vi "信号处理素材.vi"() -> ()   [LabVIEW 2018]
uses:
  <vilib>/Analysis/2dsp.llb/Upsample (DBL).vi
  <vilib>/Analysis/3filter.llb/Equi-Ripple LowPass (DBL).vi
  <vilib>/Analysis/NI_AALBase.lvlib
  <vilib>/Analysis/NI_AALPro.lvlib
panel:
  out "波形图 7":T1(graph)
  out "波形图 6":dbl[](graph)
  in  "sampling freq: fs":dbl=1.0 caption="采样频率:fs" format="%0.2f"
  in  "stop freq":dbl=0.25 caption="阻带截止频率" format="%0.2f"
  in  "pass freq":dbl=0.2 caption="通带截止频率" format="%0.2f"
  out "波形图 5":T1(graph)
  out "波形图 4":dbl[](graph)
  in  "upsampling factor":i32=1 caption="升采样因子"
  out "波形图 3":T1(graph)
  out "波形图 2":dbl[](graph)
  out "phase out":dbl caption="相位输出" format="%0.2e"
  in  "phase in":dbl caption="相位输入" format="%0.2f"
  in  "duty cycle (%)":dbl=50.0 caption="占空比(%)" format="%0.2f"
  in  "frequency":dbl=0.0078125 caption="频率" format="%.4f"
  in  "amplitude 3":dbl=1.0 caption="幅值" format="%0.2f"
  in  "samples 3":i32=128 caption="采样"
  in  "samples 2":i32=128 caption="采样"
  in  "amplitude 2":dbl=1.0 caption="幅值" format="%0.2f"
  out "波形图":dbl[](graph)
  in  "samples":i32=128 caption="采样"
  in  "amplitude":dbl=1.0 caption="幅值" format="%0.2f"
  in  "phase(degrees)":dbl caption="相位（度）" format="%0.2f"
  in  "cycles":dbl=1.0 caption="周期" format="%0.2f"
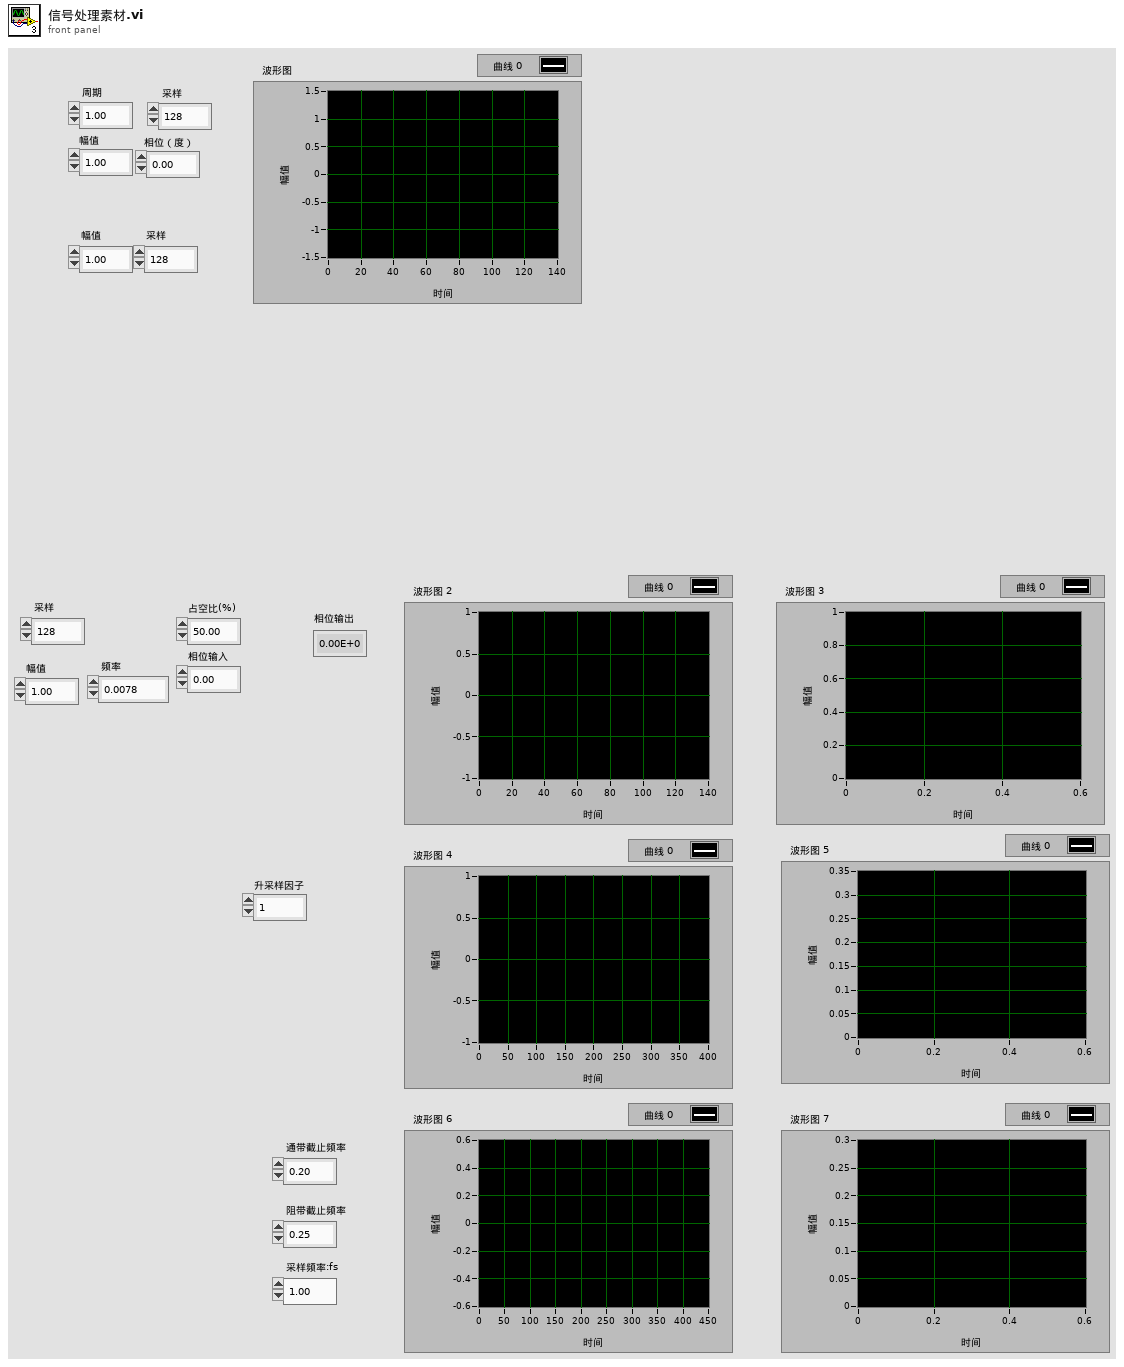
[diagram p1: front panel]
types:
  T1 = cluster{i32, "df":dbl, "Amp Spectrum Mag (Vrms)":dbl[]}
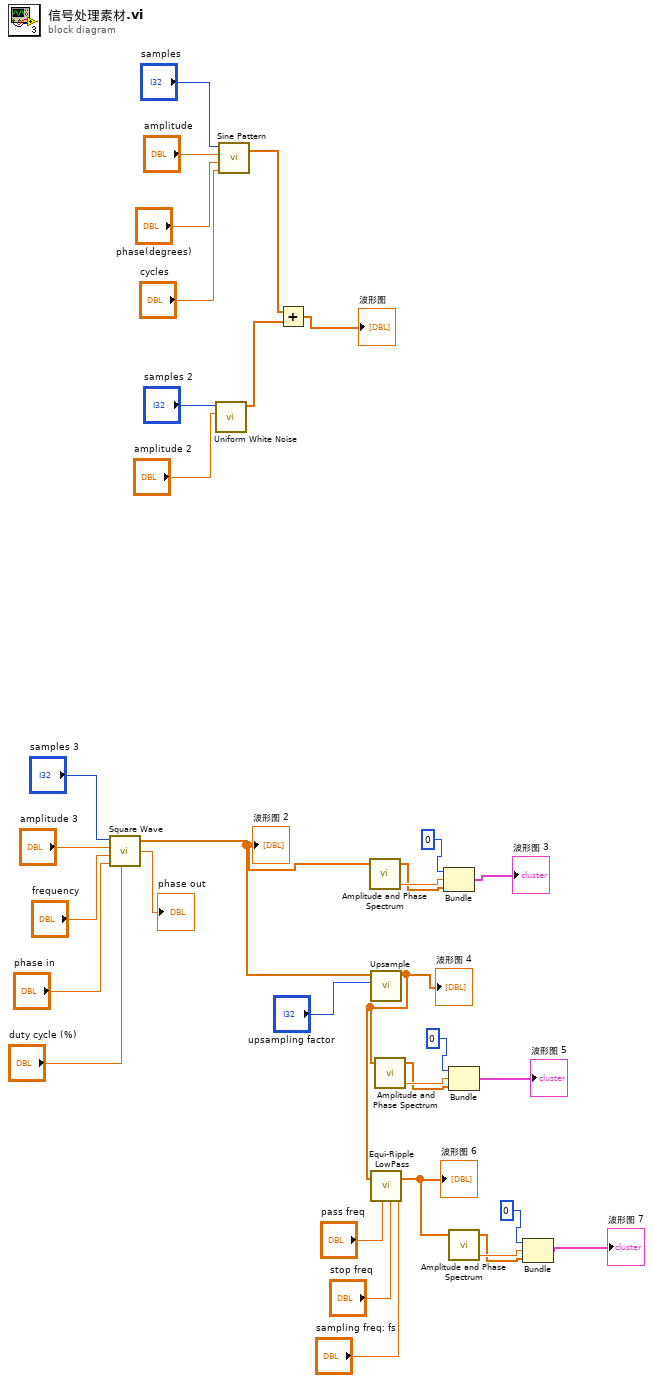
[diagram p0: block diagram]
diagram:
  n1 = call <vilib>:"Square Wave.vi"("samples"="samples 3", "amplitude"="amplitude 3", "frequency"="frequency", "duty cycle (%)"="duty cycle (%)", "phase in"="phase in") -> ("square wave"=w15:dbl[], "phase out"=→"phase out":dbl)  [unwired: 1 in, 1 out]
  "波形图 2" <- w15
  n2 = call <vilib>:"Uniform White Noise.vi"("amplitude"="amplitude 2", "samples"="samples 2") -> ("uniform white noise"=w28:dbl[])  [unwired: 8 in, 1 out]
  n3 = call <vilib>:"Sine Pattern.vi"("cycles"="cycles", "phase(degrees)"="phase(degrees)", "amplitude"="amplitude", "samples"="samples") -> ("Sinusoidal Pattern"=w27:dbl[])  [unwired: 1 out]
  n4 = Add(x=w27, y=w28) -> (x+y=→"波形图":dbl[])
  n5 = call <vilib>:"Amplitude and Phase Spectrum.vi"("Signal (V)"=w15) -> ("df"=w18:dbl, "Amp Spectrum Mag (Vrms)"=w17:dbl[])  [unwired: 2 in, 1 out]
  n6 = call-poly <vilib>:"Upsample.vi"("upsampling factor"="upsampling factor", "X"=w15) -> ("Upsampled Array"=w9:dbl[])  [unwired: 8 in, 1 out]
  "波形图 4" <- w9
  n7 = call-poly <vilib>:"Equi-Ripple LowPass.vi"("pass freq"="pass freq", "stop freq"="stop freq", "sampling freq: fs"="sampling freq: fs", "X"=w9) -> ("Filtered X"=w2:dbl[])  [unwired: 2 in, 1 out]
  "波形图 6" <- w2
  n8 = call <vilib>:"Amplitude and Phase Spectrum.vi"("Signal (V)"=w9) -> ("df"=w12:dbl, "Amp Spectrum Mag (Vrms)"=w11:dbl[])  [unwired: 2 in, 1 out]
  n9 = Bundle(0, "df"=w18, "Amp Spectrum Mag (Vrms)"=w17) -> (→"波形图 3":T1)  [unwired: 1 in]
  n10 = Bundle(0, "df"=w12, "Amp Spectrum Mag (Vrms)"=w11) -> (→"波形图 5":T1)  [unwired: 1 in]
  n11 = call <vilib>:"Amplitude and Phase Spectrum.vi"("Signal (V)"=w2) -> ("df"=w4:dbl, "Amp Spectrum Mag (Vrms)"=w3:dbl[])  [unwired: 2 in, 1 out]
  n12 = Bundle(0, "df"=w4, "Amp Spectrum Mag (Vrms)"=w3) -> (→"波形图 7":T1)  [unwired: 1 in]
